vi "NNPC_Extract_Bad_Pixel_Scores.vi"(5 "Extract Good Pixels from Bad Images":bool, 6 "Test Dataset":T1, 8 "error in":errorcluster, 10 "Bad Pixel Scores":sgl[][][](array[numeric]), 11 "Good Pixel Scores":sgl[][][](array[numeric])) -> (0 "error out":errorcluster, 2 "Bad Pixel Scores":sgl[](array[numeric]), 3 "Good Pixel Scores":sgl[](array[numeric]))   [LabVIEW 2020]
uses:
  <vilib>/Ngene/Deep Learning Toolkit/Toolkit/NN_Data/API/DataSet/DataSet_Types/NN_DataSet(In3D_Out3D).ctl
  <vilib>/Ngene/Deep Learning Toolkit/Toolkit/NN_Data/API/NN_Dims(C,H,W).ctl
  <vilib>/Ngene/Deep Learning Toolkit/Toolkit/NN_Data/Controls/DataRef_Types/4D/NN_Data_ref(4D_SGL).ctl
  <vilib>/Ngene/Deep Learning Toolkit/Toolkit/Deep_Learning_Toolkit_by_Ngene.lvlib
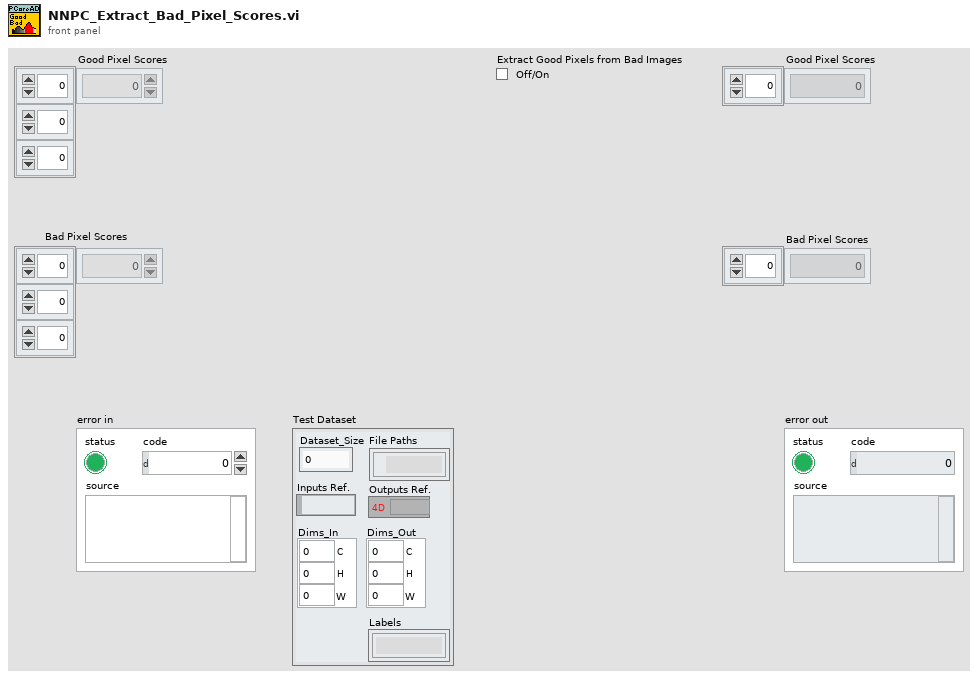
[diagram p1: front panel]
types:
  T1 = typedef "Deep_Learning_Toolkit_by_Ngene.lvlib/NN_DataSet(In3D_Out3D).ctl" = cluster{"Dataset_Size":i32, "Dims_In":T2, "Labels":string[], "File Paths":path[], "Outputs Ref.":T3, "Inputs Ref.":variant, "Dims_Out":T2}
  T2 = typedef "Deep_Learning_Toolkit_by_Ngene.lvlib/NN_Dims(C,H,W).ctl" = cluster{"C":i32, "H":i32, "W":i32}
  T3 = typedef "Deep_Learning_Toolkit_by_Ngene.lvlib/NN_Data_ref(4D_SGL).ctl" = refnum<data-value>
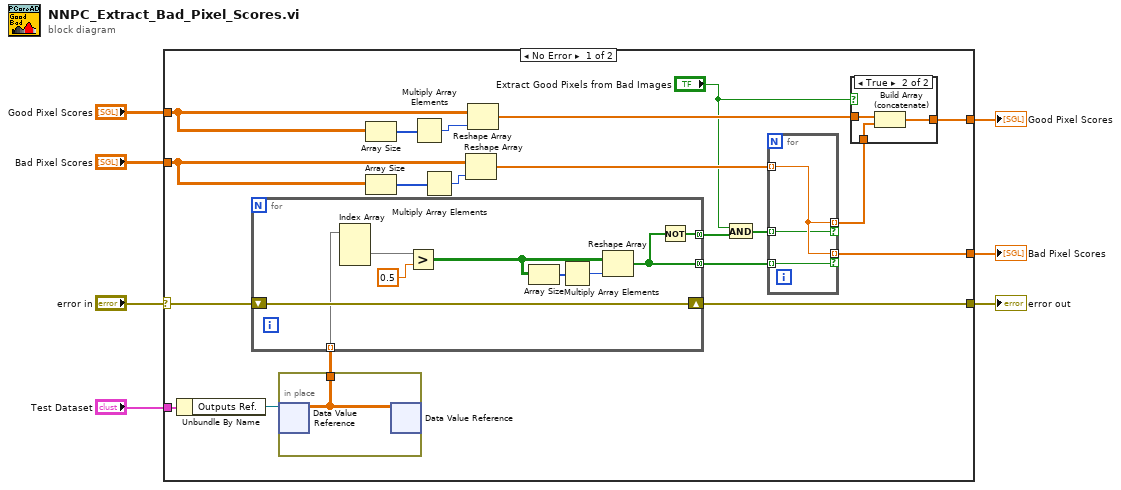
[diagram p0: block diagram]
diagram:
  n1 = case shown="No Error" "error in" {
    selector: "error in" -> [w23 w45]
    tunnel: [w27 w45] -> w7
    tunnel: [w25 _] -> w6
    tunnel: [w24 _] -> w5
    tunnel: "Good Pixel Scores" -> [w20 _]
    tunnel: "Bad Pixel Scores" -> [w13 _]
    tunnel: "Test Dataset" -> [w10 _]
    frame No Error {
      n2 = Unbundle By Name(w10) -> ("Outputs Ref."=w12:T3)
      n3 = in-place {
        in-place-border: [w44] -> w11
        n4 = in-place-dvr #1(w12) -> (w44:sgl[][][][])  [unwired: 1 out]
        n5 = in-place-dvr #1(w44) -> ()  [unwired: 2 out]
      }
      n6 = for {
        shift-right: [w42] -> w27
        shift-left: w23 -> [w42]
        tunnel: [w40] -> w14 mode=concatenating
        tunnel: [w35] -> w15 mode=concatenating
        tunnel: w11 -> [w39] mode=indexing
        n7 = Index Array(array=w39) -> (element=w38:sgl[][])  [unwired: 3 in]
        n8 = Greater?(x=w38, y=sgl 0.5) -> (0:w36:bool[][])
        n9 = Array Size(array=w36) -> (size(s)=w43:i32[])
        n10 = Multiply Array Elements(1:w43) -> (0:w41:i32)
        n11 = Reshape Array(w36, w41) -> (w35:bool[])
        n12 = Not(x=w35) -> (.not. x?=w40:bool[])
      }
      n13 = Array Size(array=w20) -> (size(s)=w19:i32[])
      n14 = Array Size(array=w13) -> (size(s)=w17:i32[])
      n15 = Multiply Array Elements(1:w19) -> (0:w18:i32)
      n16 = Multiply Array Elements(1:w17) -> (0:w16:i32)
      n17 = Reshape Array(w13, w16) -> (w22:sgl[])
      n18 = Reshape Array(w20, w18) -> (w21:sgl[])
      n19 = And(x="Extract Good Pixels from Bad Images", y=w14) -> (x .and. y?=w9:bool[])
      n20 = for {
        tunnel: w22 -> [w34] mode=indexing
        tunnel: w9 -> [w33] mode=indexing
        tunnel: w15 -> [w32] mode=indexing
        tunnel: [w34] -> w26 mode=indexing if=w33
        tunnel: [w34] -> w25 mode=indexing if=w32
      }
      n21 = case shown="True" "Extract Good Pixels from Bad Images" {
        tunnel: w21 -> [w28 w31]
        tunnel: w26 -> [_ w30]
        tunnel: [w28 w29] -> w24
        frame False {
        }
        frame True {
          n22 = Build Array (concatenate)(w31, w30) -> (w29:sgl[])
        }
      }
    }
    frame Error {
    }
  }
  "Good Pixel Scores" <- w5
  "Bad Pixel Scores" <- w6
  "error out" <- w7
